vi "GetExposureTime.vi"(1 "ModelEditInfo":T1) -> (0 "曝光时间":cluster{"[0]":i32, "[1]":i32})   [LabVIEW 2014]
uses:
  ModelEditSubVIs/ModeEditeControl.ctl
  ModelEditSubVIs/ModelInforItem.ctl
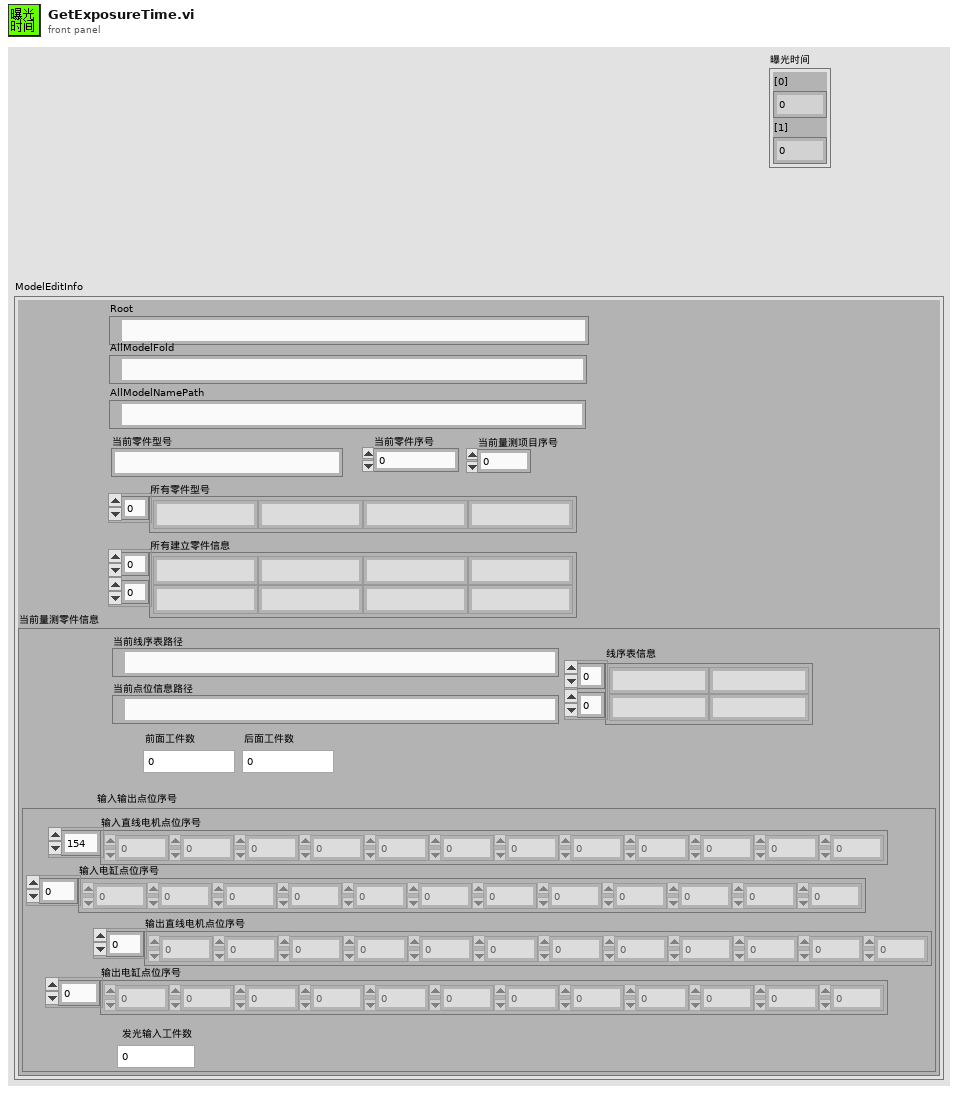
[diagram p1: front panel]
types:
  T1 = typedef "ModeEditeControl.ctl" = cluster{"Root":path, "AllModelFold":path, "AllModelNamePath":path, "所有零件型号":string[], "当前零件型号":string, "所有建立零件信息":string[][], "当前零件序号":i32, "当前量测项目序号":i32, "当前量测零件信息":cluster{"当前点位信息路径":path, "当前线序表路径":path, "输入输出点位序号":T2, "线序表信息":string[][], "前面工件数":i32, "后面工件数":i32}}
  T2 = typedef "输入输出点位序号.ctl" = cluster{"输入直线电机点位序号":i32[], "输入电缸点位序号":i32[], "输出直线电机点位序号":i32[], "输出电缸点位序号":i32[], " 发光输入工件数":i32}
  T3 = typedef "ModelInforItem.ctl" = enum16{"零件编号", "线序表地址", "前面工件数", "相机1曝光时间", "相机2曝光时间", "自动抛料"}
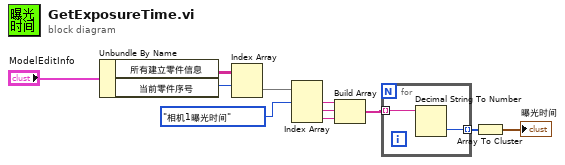
[diagram p0: block diagram]
diagram:
  n1 = Unbundle By Name("ModelEditInfo") -> ("所有建立零件信息"=w3:string[][], "当前零件序号"=w2:i32)
  n2 = Index Array(array=w3, index (row)=w2) -> (element=w4:string[])  [unwired: 1 in]
  n3 = Index Array(array=w4, index #1=ModelInforItem."相机1曝光时间" ("零件信息项目名称")) -> (element #1=w6:string, element #2=w7:string, element #3=w8:string)  [unwired: 2 in]
  n4 = Build Array(w6, w7, w8) -> (w10:string[])
  n5 = for {
    tunnel: w10 -> [w13] mode=indexing
    tunnel: [w12] -> w11 mode=indexing
    n6 = Decimal String To Number(string=w13) -> (number=w12:i32)  [unwired: 2 in, 1 out]
  }
  n7 = Array To Cluster(array=w11) -> (cluster=→"曝光时间":cluster{"[0]":i32, "[1]":i32})
